vi "Random with Probability.vi"(11 "Probability":dbl[](array[numeric])) -> (3 "Class":i32)   [LabVIEW 2014, in "HMM.lvlib"]
doc: "Generates a random class based on the input probability. \n\nE.g. the input probabilities are [0.5, 0.3, 0.2] then Pr(0) = 0.5, Pr(1) = 0.3, Pe(2) = 0.2."
uses:
  HMM.lvlib
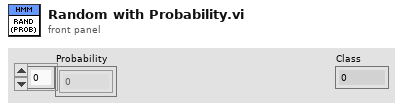
[diagram p1: front panel]
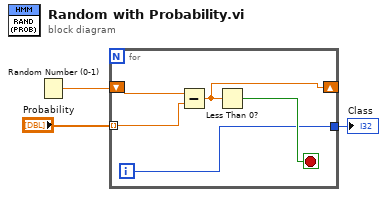
[diagram p0: block diagram]
diagram:
  n1 = Random Number (0-1)() -> (number: 0 to 1=w2:dbl)
  n2 = for {
    tunnel: "Probability" -> [w8] mode=indexing
    tunnel: [w6] -> w1
    shift-right: [w4] -> _
    shift-left: w2 -> [w5]
    i -> [w6]
    stop <- w7 stop-if-true
    n3 = Subtract(x=w5, y=w8) -> (x-y=w4:dbl)
    n4 = Less Than 0?(x=w4) -> (x < 0?=w7:bool)
  }
  "Class" <- w1
